vi "getMessage.vi"(8 "error in (no error)":errorcluster, 11 "Communicator in":refnum<class "Communicator.lvclass">) -> (0 "error out":errorcluster, 2 "String":string, 3 "Communicator out":refnum<class "Communicator.lvclass">)   [LabVIEW 2016, in "Communicator.lvclass"]
uses:
  Communicator.lvclass
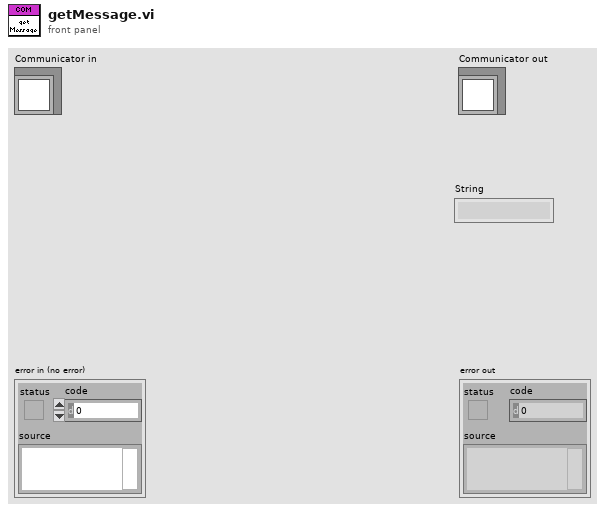
[diagram p1: front panel]
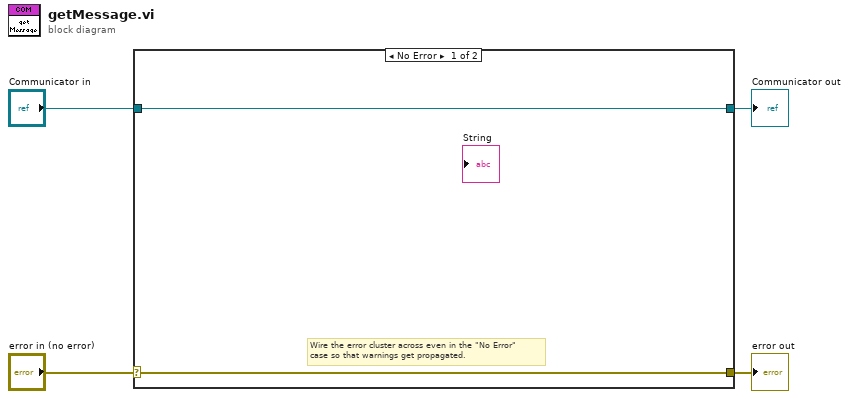
[diagram p0: block diagram]
diagram:
  n1 = case shown="No Error" "error in (no error)" {
    selector: "error in (no error)" -> [w5 w8]
    tunnel: [w5 w8] -> w3
    tunnel: [w6 w7] -> w1
    tunnel: "Communicator in" -> [w6 w7]
    frame No Error {
      # "Wire the error cluster across even in the \"No Error\"\ncase so that warnings get propagated."
    }
    frame Error {
    }
  }
  "error out" <- w3
  "Communicator out" <- w1
